vi "BUCK_ESO_SMC_finalversion.vi"() -> ()   [LabVIEW 2018]
doc: "I. Description:\nThis example demonstrates how to continuously output a waveform using an internal sample clock. The automatic regeneration of data has been disabled, so new data has to be provided throughout the duration of the continuous Analog Output operation. This allows the generation of any arbitrary frequency as this VI computes new data for each iteration of the loop, maintaining phase continuity of the signal.\n\nII. Instructions for Running:\n1. Select the Physical Channel to correspond to where your signal is output on the DAQ device.\n2. Enter the Minimum and Maximum Voltage range.\n3. Specify the desired Sample Clock Rate of the output Waveform. Higher sample clock rates will produce a smoother waveform.\n4. Manually specify the Analog Output buffer size, in number of samples. A larger buffer would help non-regenerative operations avoid errors due to occasional high CPU load. \nNote: \nThe Analog Output buffer has to be at least as big as the amount of data being written to the board per iteration. The recommended buffer size would be at least twice the amount of data being written to the board per iteration.\n5. Enter the Waveform Information. See the documentation of the Basic Function Generator SubVI for information on each parameter.\n\nIII. Block Diagram Steps:\n1. Create an Analog Output Voltage channel.\n2. Configure the task to prohibit the automatic regeneration of data.\n3. Call the DAQmx (Sample Clock) VI to set the sample clock rate. Additionally, set the sample mode to Continuous.\n4. Read the actual sample clock rate (eventually coerced depending on the hardware used). \n5. Compute the desired waveform, using the buffer size and the actual update rate. This VI keeps track of the phase of the waveform to ensure that the generated signal is continuous.\n6. Write the waveform to the output buffer. \n7a. Call the Start VI. This is only needed when the loop is executed for the first time.\n7b. Do nothing.\n8. Loop continuously until user presses the Stop button. Every iteration computes and writes a new waveform to the buffer.\n9. Call the Clear Task VI to clear the Task.\n10. Use the popup dialog box to display an error or warning if any.\n\nIV. I/O Connections Overview:\nMake sure your signal output terminal matches the Physical Channel I/O Control. For further connection information, refer to your hardware reference manual."
uses:
  <vilib>/Utility/error.llb/DialogType.ctl
  <vilib>/Analysis/8numeric.llb/1D Numeric Integration.vi
  <vilib>/DAQmx/read.llb/DAQmx Read (Analog 1D DBL NChan 1Samp).vi
  <vilib>/DAQmx/write.llb/DAQmx Write (Analog 1D DBL 1Chan NSamp).vi
  <vilib>/DAQmx/create/channels.llb/DAQmx Create Channel (AO-Voltage-Basic).vi
  <vilib>/DAQmx/configure/timing.llb/DAQmx Timing (Sample Clock).vi
  <vilib>/DAQmx/create/channels.llb/DAQmx Create Channel (AI-Voltage-Basic).vi
  <vilib>/DAQmx/miscellaneous.llb/DAQmx Fill In Error Info.vi
  <resource>/objmgr/daqmx.rc
  <vilib>/measure/NI_MABase.lvlib
  <vilib>/Analysis/NI_AALPro.lvlib
panel:
  in  "s":bool=TRUE
  out "real占空比":dbl(graph)=0.7177033492822967
  in  "Vin":dbl=16.72
  in  "Vr":dbl
  in  "test占空比":dbl=1.0
  in  "dt":dbl=0.1
  in  "Sample Clock Rate 2":dbl=10.0 format="%0.2f"
  out "x1":dbl(graph)=-0.06980003427729287
  out "eta_sgn":dbl(graph)=1000.0
  out "d1_hat":dbl(graph)=1062.5619418417389
  out "x2":dbl(graph)=-468.07395564625267
  out "z1-x1":dbl(graph)=146.86982957294958
  in  "k":dbl=10.0
  in  "beta2":dbl=100.0
  in  "beta1":dbl=20.0
  in  "eta":dbl=1000.0
  in  "R0":dbl=20.0
  in  "L0":dbl=0.01
  in  "C0":dbl=0.001
  out "Vout":dbl(graph)=11.930199965722707
  out "VSM025A":dbl(graph)=0.3304106319556013
  out "CSM025A":dbl(graph)=0.3018247002037242
  in  "offset":dbl=0.5 caption="偏移量" format="%0.2p"
  in  "Maximum Value 3":dbl=10.0 caption="Maximum Value" format="%0.2f"
  in  "Minimum Value 3":dbl=-10.0 caption="Minimum Value" format="%0.2f"
  in  "Samples per Channel 2":i32=10000 caption="Samples per Channel"
  in  "Physical Channel 2":tag="myDAQ1/ai0:1"
  out "占空比":dbl(graph)=0.6659410304297767
  in  "Size (Samples)":u32=10000
  out "Actual Sample Clock Rate":dbl=100000.0 format="%.2f"
  in  "Sample Clock Rate":dbl=100000.0 format="%0.2f"
  in  "Waveform Type":T1(ring)=enum."Triangle Wave"
  in  "Frequency":dbl=4500.0 format="%.2f"
  in  "Amplitude":dbl=0.5 format="%0.2p"
  out "Waveform Graph":waveform(dbl)(graph)={"t0"=timestamp(19.6 s since 1904-01-01), "dt"=1e-05, "Y"=[]} caption="Output Waveform"
  in  "Physical Channels":tag="myDAQ1/ao0"
  in  "Minimum Value":dbl=-10.0 format="%0.2f"
  in  "Maximum Value":dbl=10.0 format="%0.2f"
  in  "stop":bool
  # "Channel Parameters"
  # "Timing Parameters"
  # "Buffer Parameters"
  # "Waveform Information"
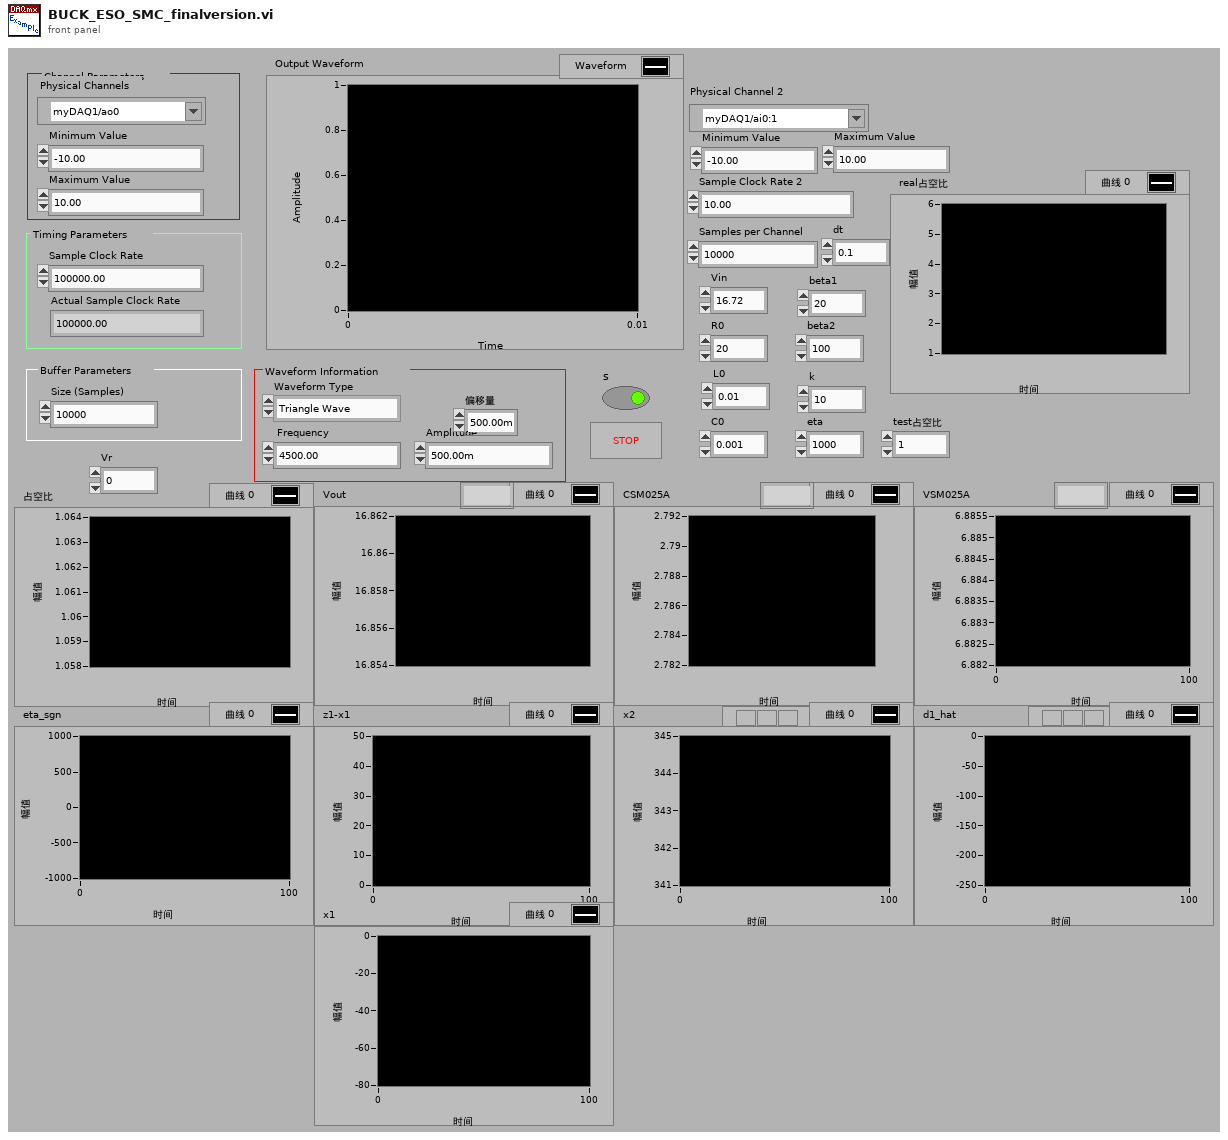
[diagram p1: front panel]
types:
  T1 = enum16{"Sine Wave", "Triangle Wave", "Square Wave", "Sawtooth Wave"}
  T2 = typedef "DialogType.ctl" = u16
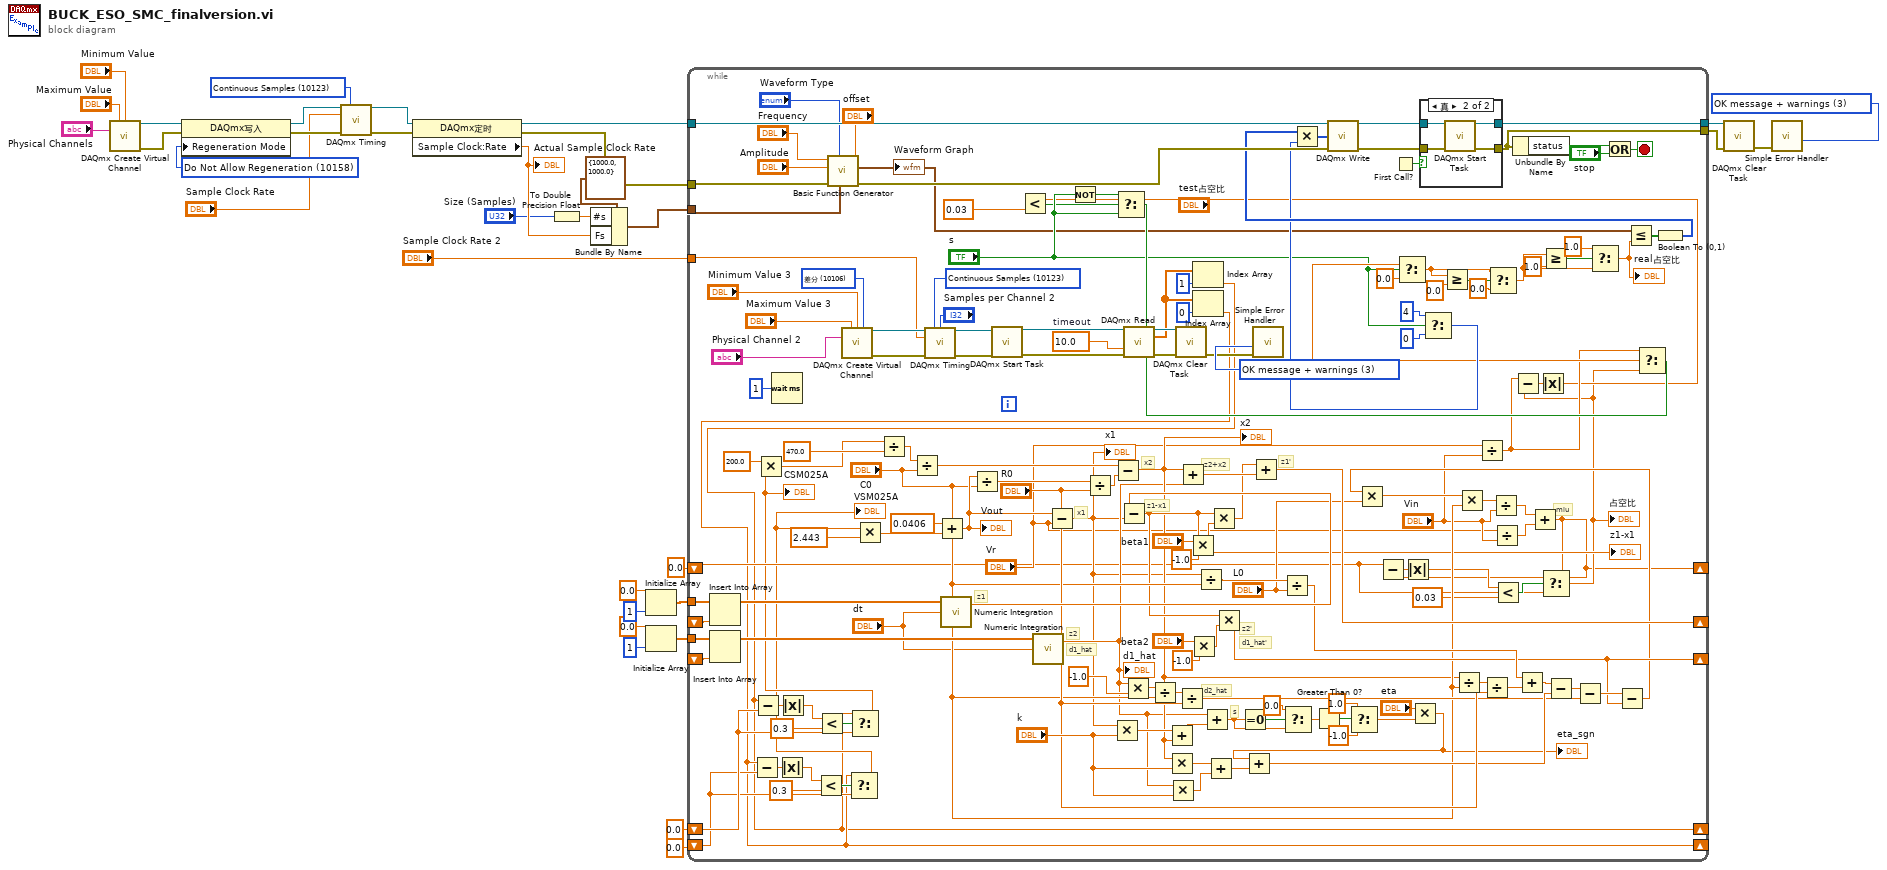
[diagram p0: block diagram]
diagram:
  w20 = 10158 items=["Allow Regeneration"=10097, "Do Not Allow Regeneration"=10158] ("RegenMode")
  w28 = T2 3 items=["no dialog", "OK message", "continue or stop message", "OK message + warnings", "continue/stop + warnings"] ("type of dialog (OK msg:1)")
  w32 = 10123 items=["Finite Samples"=10178, "Continuous Samples"=10123] ("sample mode")
  n1 = call-poly <vilib>:"DAQmx Create Virtual Channel.vi"("maximum value"="Maximum Value", "minimum value"="Minimum Value", "physical channels"="Physical Channels") -> ("task out"=w19:refnum<k21>, "error out"=w18:errorcluster)  [unwired: 11 in]
  n2 = property class="DAQmx写入"(reference=w19, error in=w18, "Regeneration Mode"=w20) -> (reference out=w13:refnum<k21>, error out=w12:errorcluster)
  n3 = call-poly <vilib>:"DAQmx Timing.vi"("task/channels in"=w13, "sample mode"=w32, "rate"="Sample Clock Rate", "error in"=w12) -> ("task out"=w25:refnum<k21>, "error out"=w24:errorcluster)  [unwired: 10 in]
  n4 = property class="DAQmx定时"(reference=w25, error in=w24) -> (reference out=w17:refnum<k21>, error out=w16:errorcluster, "Sample Clock:Rate"=w22:dbl)
  "Actual Sample Clock Rate" <- w22
  n5 = To Double Precision Float(number="Size (Samples)") -> (double precision float=w14:dbl)
  n6 = Bundle By Name(cluster=cluster{"Fs":dbl, "#s":dbl} {"Fs"=1000.0, "#s"=1000.0} ("sampling info"), "#s"=w14, "Fs"=w22) -> (w21:cluster{"Fs":dbl, "#s":dbl})
  n7 = Initialize Array(0.0 ("元素"), 1 ("维数大小")) -> (w5:dbl[])
  n8 = Initialize Array(0.0 ("元素"), 1 ("维数大小")) -> (w6:dbl[])
  n9 = while {
    tunnel: w17 -> [w184]
    tunnel: [w181] -> w27
    tunnel: w16 -> [w172]
    tunnel: [w173] -> w26
    tunnel: w21 -> [w185]
    tunnel: "Sample Clock Rate 2" -> [w156]
    shift-right: [w124] -> _
    shift-left: _ -> [w123]
    shift-right: [w86] -> _
    shift-left: _ -> [w118]
    tunnel: w6 -> [w76]
    tunnel: w5 -> [w75]
    shift-right: [w50] -> _
    shift-left: 0.0 ("元素") -> [w49]
    shift-right: [w35] -> _
    shift-left: 0.0 ("元素") -> [w38]
    shift-right: [w36] -> _
    shift-left: 0.0 ("元素") -> [w37]
    stop <- w189 stop-if-true
    w154 = 10106 items=["默认"=-1, "RSE"=10083, "NRSE"=10078, "差分"=10106, "伪差分"=12529] ("input terminal configuration")
    w158 = T2 3 items=["no dialog", "OK message", "continue or stop message", "OK message + warnings", "continue/stop + warnings"] ("type of dialog (OK msg:1)")
    w171 = 10123 items=["Finite Samples"=10178, "Continuous Samples"=10123] ("sample mode")
    w174 = 10.0  # timeout
    # "miu"
    # "s"
    # "d2_hat"
    # "d1_hat'"
    # "d1_hat"
    # "z2"
    # "z2'"
    # "z2+x2"
    # "z1-x1"
    # "z1"
    # "z1'"
    # "x1"
    # "x2"
    n10 = Insert Into Array(array=w75, new element=w123) -> (w130:dbl[])  [unwired: 1 in]
    n11 = Insert Into Array(array=w76, new element=w118) -> (w119:dbl[])  [unwired: 1 in]
    n12 = Wait (ms)(milliseconds to wait=u32 1 ("等待时间（毫秒）")) -> ()  [unwired: 1 out]
    n13 = call <vilib>:"Basic Function Generator.vi"("offset"="offset", "sampling info"=w185, "signal type"="Waveform Type", "error in (no error)"=w172, "amplitude"="Amplitude", "frequency"="Frequency") -> ("error out"=w186:errorcluster, "signal out"=w61:waveform(dbl))  [unwired: 3 in, 1 out]
    "Waveform Graph" <- w61
    n14 = call-poly <vilib>:"DAQmx Create Virtual Channel.vi"("maximum value"="Maximum Value 3", "minimum value"="Minimum Value 3", "input terminal configuration"=w154, "physical channels"="Physical Channel 2") -> ("task out"=w169:refnum<k21>, "error out"=w167:errorcluster)  [unwired: 10 in]
    n15 = call-poly <vilib>:"DAQmx Timing.vi"("task/channels in"=w169, "sample mode"=w171, "samples per channel"="Samples per Channel 2", "rate"=w156, "error in"=w167) -> ("task out"=w164:refnum<k21>, "error out"=w163:errorcluster)  [unwired: 9 in]
    n16 = call-poly <vilib>:"Numeric Integration.vi"("dt"="dt", "Input Array"=w130) -> ("result"=w129:dbl)  [unwired: 1 in, 1 out]
    n17 = call <vilib>:"DAQmx Start Task.vi"("task/channels in"=w164, "error in"=w163) -> ("task out"=w162:refnum<k21>, "error out"=w161:errorcluster)  [unwired: 12 in]
    n18 = call-poly <vilib>:"Numeric Integration.vi"("dt"="dt", "Input Array"=w119) -> ("result"=w72:dbl)  [unwired: 1 in, 1 out]
    "d1_hat" <- w72
    n19 = Not(x="s") -> (.not. x?=w66:bool)
    n20 = Multiply(x=w72, y=-1.0) -> (x*y=w116:dbl)
    n21 = call-poly <vilib>:"DAQmx Read.vi"("task/channels in"=w162, "timeout"=w174, "error in"=w161) -> ("task out"=w160:refnum<k21>, "data"=w139:dbl[], "error out"=w159:errorcluster)  [unwired: 10 in]
    n22 = Divide(x=w116, y="C0") -> (x/y=w115:dbl)
    n23 = Multiply(x=w72, y="k") -> (x*y=w100:dbl)
    n24 = call <vilib>:"DAQmx Clear Task.vi"("task in"=w160, "error in"=w159) -> ("error out"=w157:errorcluster)  [unwired: 13 in]
    n25 = Divide(x=w115, y="R0") -> (x/y=w85:dbl)
    n26 = Multiply(x="beta1", y=-1.0) -> (x*y=w127:dbl)
    n27 = Multiply(x="beta2", y=-1.0) -> (x*y=w120:dbl)
    n28 = Index Array(array=w139, index=1 ("索引")) -> (element=w35:dbl)
    n29 = Subtract(x=w35, y=w38) -> (x-y=w48:dbl)
    n30 = Absolute Value(x=w48) -> (abs(x)=w46:dbl)
    n31 = Less?(x=w46, y=0.3) -> (x < y?=w45:bool)
    n32 = Select(t=w35, s=w45, f=w38) -> (s? t:f=w40:dbl)
    "CSM025A" <- w40
    n33 = Multiply(x=200.0, y=w40) -> (x*y=w96:dbl)
    n34 = Divide(x=w96, y=470.0 ("x")) -> (x/y=w99:dbl)
    n35 = Divide(x=w99, y="C0") -> (x/y=w135:dbl)
    n36 = Index Array(array=w139, index=0 ("索引")) -> (element=w36:dbl)
    n37 = Subtract(x=w36, y=w37) -> (x-y=w44:dbl)
    n38 = Absolute Value(x=w44) -> (abs(x)=w42:dbl)
    n39 = Less?(x=w42, y=0.3) -> (x < y?=w41:bool)
    n40 = Select(t=w36, s=w41, f=w37) -> (s? t:f=w39:dbl)
    "VSM025A" <- w39
    n41 = Multiply(x=w39, y=2.443) -> (x*y=w137:dbl)
    n42 = Add(x=0.0406, y=w137) -> (x+y=w134:dbl)
    "Vout" <- w134
    n43 = Divide(x=w134, y="C0") -> (x/y=w133:dbl)
    n44 = Subtract(x=w134, y="Vr") -> (x-y=w70:dbl)
    "x1" <- w70
    n45 = Divide(x=w133, y="R0") -> (x/y=w132:dbl)
    n46 = Multiply(x=w70, y="k") -> (x*y=w114:dbl)
    n47 = Subtract(x=w135, y=w132) -> (x-y=w73:dbl)
    "x2" <- w73
    n48 = Subtract(x=w129, y=w70) -> (x-y=w74:dbl)
    "z1-x1" <- w74
    n49 = Add(x=w114, y=w73) -> (x+y=w113:dbl)
    n50 = Multiply(x=w73, y="k") -> (x*y=w101:dbl)
    n51 = Add(x=w73, y=w72) -> (x+y=w131:dbl)
    n52 = Divide(x=w70, y="C0") -> (x/y=w95:dbl)
    n53 = Add(x=w72, y=w113) -> (x+y=w111:dbl)
    n54 = Add(x=w101, y=w100) -> (x+y=w102:dbl)
    n55 = Multiply(x=w74, y=w127) -> (x*y=w125:dbl)
    n56 = Multiply(x=w74, y=w120) -> (x*y=w86:dbl)
    n57 = Equal To 0?(x=w111) -> (x = 0?=w112:bool)
    n58 = Add(x=w125, y=w131) -> (x+y=w124:dbl)
    n59 = call <vilib>:"Simple Error Handler.vi"("type of dialog (OK msg:1)"=w158, "error in (no error)"=w157) -> ()  [unwired: 3 in, 5 out]
    n60 = Divide(x=w95, y="L0") -> (x/y=w90:dbl)
    n61 = Select(t=0.0, s=w112, f=w111) -> (s? t:f=w109:dbl)
    n62 = Greater Than 0?(x=w109) -> (x > 0?=w108:bool)
    n63 = Select(t=1.0, s=w108, f=-1.0) -> (s? t:f=w105:dbl)
    n64 = First Call?() -> (First Call?: T/F=w180:bool)
    n65 = Multiply(x="eta", y=w105) -> (x*y=w71:dbl)
    "eta_sgn" <- w71
    n66 = Add(x=w71, y=w102) -> (x+y=w88:dbl)
    n67 = Select(t=4, s="s", f=0) -> (s? t:f=w151:i32)
    n68 = Divide(x=w73, y="C0") -> (x/y=w93:dbl)
    n69 = Divide(x="Vr", y="Vin") -> (x/y=w59:dbl)
    n70 = Divide(x=w93, y="R0") -> (x/y=w89:dbl)
    n71 = Divide(x="Vr", y="Vin") -> (x/y=w78:dbl)
    n72 = Add(x=w90, y=w89) -> (x+y=w92:dbl)
    n73 = Subtract(x=w92, y=w88) -> (x-y=w91:dbl)
    n74 = Subtract(x=w91, y=w85) -> (x-y=w87:dbl)
    n75 = Subtract(x=w87, y=w86) -> (x-y=w84:dbl)
    n76 = Multiply(x=w84, y="L0") -> (x*y=w81:dbl)
    n77 = Multiply(x=w81, y="C0") -> (x*y=w80:dbl)
    n78 = Divide(x=w80, y="Vin") -> (x/y=w79:dbl)
    n79 = Add(x=w79, y=w78) -> (x+y=w50:dbl)
    n80 = Subtract(x=w49, y=w50) -> (x-y=w54:dbl)
    n81 = Absolute Value(x=w54) -> (abs(x)=w52:dbl)
    n82 = Less?(x=w52, y=0.03) -> (x < y?=w51:bool)
    n83 = Select(t=w50, s=w51, f=w49) -> (s? t:f=w55:dbl)
    "占空比" <- w55
    n84 = Subtract(x=w59, y=w55) -> (x-y=w60:dbl)
    n85 = Absolute Value(x=w60) -> (abs(x)=w57:dbl)
    n86 = Less?(x=w57, y=0.03) -> (x < y?=w56:bool)
    n87 = Select(t=w66, s=w56, f="s") -> (s? t:f=w65:bool)
    n88 = Select(t=w59, s=w65, f=w55) -> (s? t:f=w67:dbl)
    n89 = Select(t=w67, s="s", f=0.0) -> (s? t:f=w77:dbl)
    n90 = Greater Or Equal?(x=w77, y=0.0) -> (x >= y?=w147:bool)
    n91 = Select(t=w77, s=w147, f=0.0) -> (s? t:f=w142:dbl)
    n92 = Greater Or Equal?(x=w142, y=1.0) -> (x >= y?=w144:bool)
    n93 = Select(t=1.0, s=w144, f=w142) -> (s? t:f=w34:dbl)
    "real占空比" <- w34
    n94 = Less Or Equal?(x=w61, y=w34) -> (x <= y?=w176:bool[])
    n95 = Boolean To (0,1)(Boolean=w176) -> (0, 1=w175:i16[])
    n96 = Multiply(x=w175, y=w151) -> (x*y=w68:i32[])
    n97 = call-poly <vilib>:"DAQmx Write.vi"("task/channels in"=w184, "data"=w68, "error in"=w186) -> ("task out"=w183:refnum<k21>, "error out"=w182:errorcluster)  [unwired: 10 in, 1 out]
    n98 = case shown="真" w180 {
      tunnel: w183 -> [w191 w195]
      tunnel: w182 -> [w190 w194]
      tunnel: [w190 w193] -> w173
      tunnel: [w191 w192] -> w181
      frame False {
        # "7b."
      }
      frame True {
        n99 = call <vilib>:"DAQmx Start Task.vi"("task/channels in"=w195, "error in"=w194) -> ("task out"=w192:refnum<k21>, "error out"=w193:errorcluster)  [unwired: 12 in]
      }
    }
    n100 = Unbundle By Name(w173) -> ("status"=w188:bool)
    n101 = Or(x=w188, y="stop") -> (x .or. y?=w189:bool)
  }
  n102 = call <vilib>:"DAQmx Clear Task.vi"("task in"=w27, "error in"=w26) -> ("error out"=w33:errorcluster)  [unwired: 13 in]
  n103 = call <vilib>:"Simple Error Handler.vi"("type of dialog (OK msg:1)"=w28, "error in (no error)"=w33) -> ()  [unwired: 3 in, 5 out]
